vi "Update Subsystem View Refnums Map.vi"(8 "error in (no error)":errorcluster, 9 "Binding Control Refnums":refnum<vi>[](array[refnum]), 10 "Subsystem URL":refnum<k21>="\\\\localhost\\ABCDEFG\\TCU3", 11 "URL Refnum Map In":variant) -> (0 "error out":errorcluster, 2 "dup Subsystem URL":refnum<k21>="\\\\localhost\\ABCDEFG\\TCU3", 3 "URL Refnum Map Out":variant)   [LabVIEW 2024]
doc: "Adds the mapping relation between the URL and the front panel controls to the map."
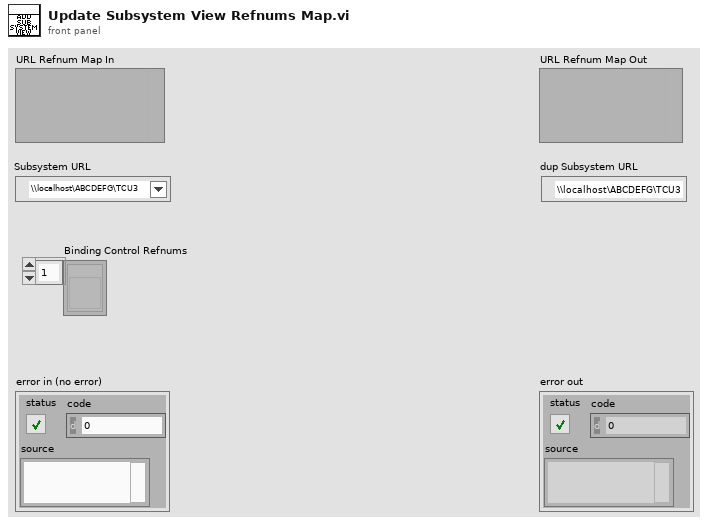
[diagram p1: front panel]
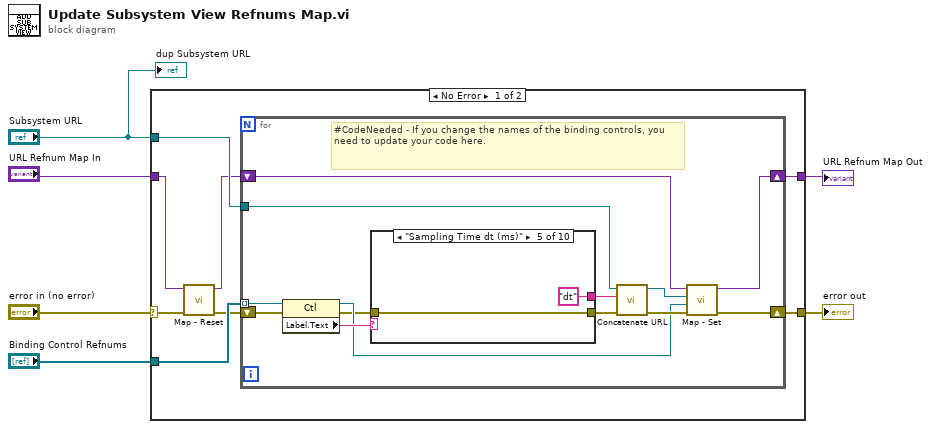
[diagram p0: block diagram]
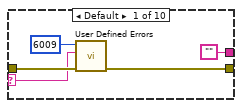
[diagram p2: hidden frame]
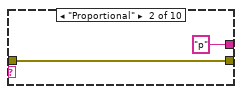
[diagram p3: hidden frame]
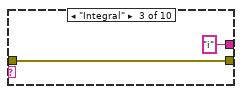
[diagram p4: hidden frame]
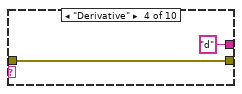
[diagram p5: hidden frame]
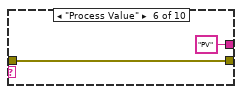
[diagram p6: hidden frame]
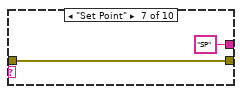
[diagram p7: hidden frame]
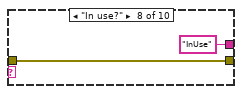
[diagram p8: hidden frame]
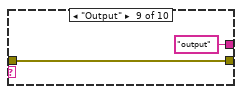
[diagram p9: hidden frame]
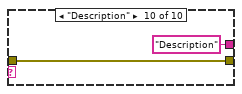
[diagram p10: hidden frame]
diagram:
  n1 = case shown="No Error" "error in (no error)" {
    selector: "error in (no error)" -> [w14 w52]
    tunnel: [w13 w52] -> w5
    tunnel: "Subsystem URL" -> [w11 _]
    tunnel: [w12 w51] -> w4
    tunnel: "URL Refnum Map In" -> [w8 w51]
    tunnel: "Binding Control Refnums" -> [w10 _]
    frame No Error {
      n2 = call "Map - Reset.vi"("error in (no error)"=w14, "Map In"=w8) -> ("error out"=w9:errorcluster, "Map Out"=w7:variant)  [unwired: 8 in]
      n3 = for {
        tunnel: w11 -> [w26]
        tunnel: w10 -> [w27] mode=indexing
        shift-right: [w23] -> w12
        shift-left: w7 -> [w25]
        shift-right: [w22] -> w13
        shift-left: w9 -> [w21]
        # "#CodeNeeded - If you change the names of the binding controls, you need to update your code here."
        n4 = property class="Ctl"(reference=w27, error in=w21) -> (reference out=w18:refnum<vi>, error out=w16:errorcluster, "Label.Text"=w20:string)
        n5 = case shown="\"Sampling Time dt (ms)\"" w20 {
          selector: w20 -> [w29 _ _ _ _ _ _ _ _ _]
          tunnel: ["" "p" "i" "d" "dt" "PV" "SP" "InUse" "output" "Description"] -> w17
          tunnel: w16 -> [w31 w33 w36 w37 w40 w41 w44 w45 w47 w49]
          tunnel: [w30 w33 w36 w37 w40 w41 w44 w45 w47 w49] -> w15
          frame Default {
            n6 = call "User Defined Errors.vi"("error in (no error)"=w31, "Parameter 1"=w29, "Error Code (0)"=6009 ("error code (0)")) -> ("error out"=w30:errorcluster)  [unwired: 8 in]
          }
          frame "Proportional" {
          }
          frame "Integral" {
          }
          frame "Derivative" {
          }
          frame "Sampling Time dt (ms)" {
          }
          frame "Process Value" {
          }
          frame "Set Point" {
          }
          frame "In use?" {
          }
          frame "Output" {
          }
          frame "Description" {
          }
        }
        n7 = call "Concatenate URL.vi"("error in (no error)"=w15, "Child Name"=w17, "Parent URL"=w26) -> ("error out"=w19:errorcluster, "Child URL"=w24:refnum<k21>)  [unwired: 7 in]
        n8 = call "Map - Set.vi"("error in (no error)"=w19, "Value"=w18, "Key"=w24, "Map In"=w25) -> ("error out"=w22:errorcluster, "Map Out"=w23:variant)  [unwired: 5 in, 1 out]
      }
    }
    frame Error {
    }
  }
  "error out" <- w5
  "URL Refnum Map Out" <- w4
  "dup Subsystem URL" <- "Subsystem URL"
